vi "DP-Append Data.vi"(0 "DataAcq":T1, 9 "Processed data":dbl[](array[numeric]), 11 "error in (no error)":errorcluster) -> (15 "error out":errorcluster)   [LabVIEW 2020]
uses:
  Typedefs/DP-Runtime State.ctl
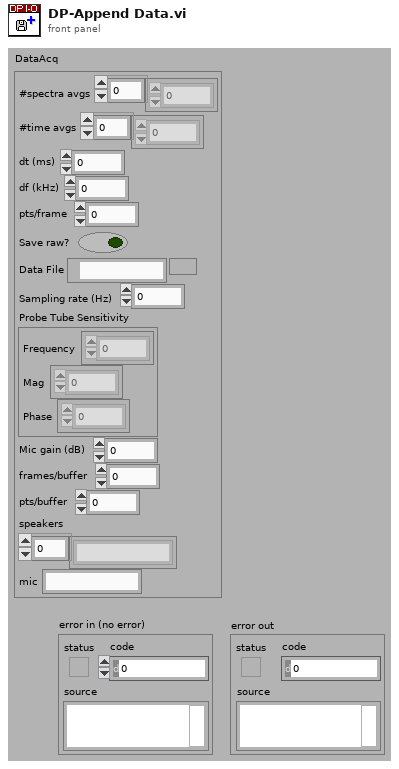
[diagram p1: front panel]
types:
  T1 = typedef "DP-Runtime State.ctl" = cluster{"#spectra avgs":i32[], "#time avgs":i32[], "dt (ms)":dbl, "df (kHz)":dbl, "pts/frame":i32, "Save raw?":bool, "Data File":path, "Sampling rate (Hz)":dbl, "Probe Tube Sensitivity":cluster{"Frequency":dbl[], "Mag":dbl[], "Phase":dbl[]}, "Mic gain (dB)":dbl, "frames/buffer":i32, "pts/buffer":i32, "speakers":string[], "mic":string}
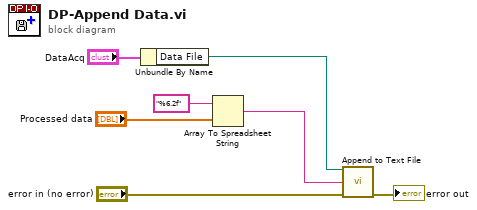
[diagram p0: block diagram]
diagram:
  n1 = Unbundle By Name("DataAcq") -> ("Data File"=w2:path)
  n2 = Array To Spreadsheet String(array="Processed data", 3:"%6.2f") -> (spreadsheet string=w1:string)  [unwired: 1 in]
  n3 = call "Append to Text File.vi"("file path"=w2, "text"=w1, "error in (no error)"="error in (no error)") -> ("error out"=→"error out":errorcluster)  [unwired: 11 in, 1 out]
